vi "invalid implementation error.vi"(8 "error in (no error)":errorcluster, 11 "params":variant) -> (0 "error out":errorcluster, 3 "data":variant)   [LabVIEW 2017]
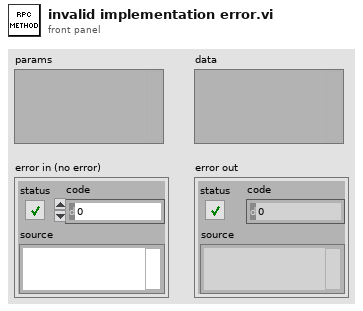
[diagram p1: front panel]
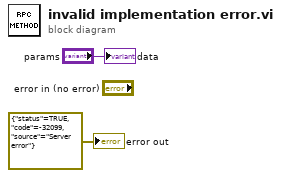
[diagram p0: block diagram]
diagram:
  "data" <- "params"
  "error out" <- errorcluster {"status"=TRUE, "code"=-32099, "source"="Server error"} ("error out")
